vi "MoveAbs_all.vi"(7 "# axis":i32, 8 "error in (no error)":errorcluster, 10 "Position":dbl[](array[numeric]), 11 "VISA resource name":refnum<visa-resource-name>) -> (0 "error out":errorcluster)   [LabVIEW 2012, in "ESP300.lvlib"]
doc: "Performs an instrument error query before terminating the software connection to the instrument."
uses:
  <instrlib>/ESP300/ESP300.lvlib
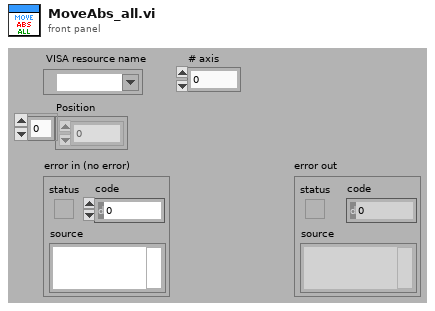
[diagram p1: front panel]
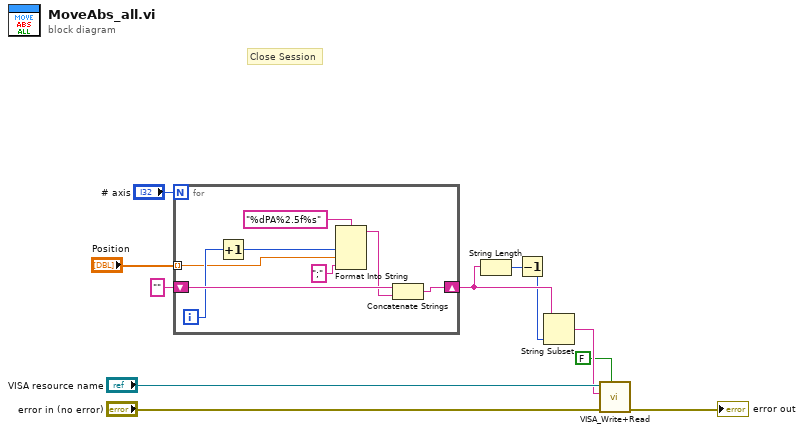
[diagram p0: block diagram]
diagram:
  # "Close Session"
  n1 = for {
    N: "# axis" -> [_]
    shift-right: [w17] -> w4
    shift-left: "" -> [w16]
    tunnel: "Position" -> [w12] mode=indexing
    i -> [w14]
    n2 = Increment(x=w14) -> (x+1=w13:i32)
    n3 = Format Into String(format string="%dPA%2.5f%s", w13, w12, ";" ("input 3")) -> (resulting string=w15:string)  [unwired: 2 in, 1 out]
    n4 = Concatenate Strings(w16, w15) -> (w17:string)
  }
  n5 = String Length(string=w4) -> (length=w3:i32)
  n6 = Decrement(x=w3) -> (x-1=w2:i32)
  n7 = String Subset(string=w4, length (rest)=w2) -> (substring=w5:string)  [unwired: 1 in]
  n8 = call <instrlib>:"VISA_Write+Read.vi"("Read?"=FALSE, "error in (no error)"="error in (no error)", "Write Buffer"=w5, "VISA resource name"="VISA resource name") -> ("error out"=→"error out":errorcluster)  [unwired: 5 in, 2 out]
